vi "display_michelle_visjitter_stopadded_RandCont_PsuedoCO_TSLogFC2.vi"() -> ()   [LabVIEW 2019]
uses:
  <vilib>/Analysis/Matrix/Datatypes/RealMatrix.ctl
  <vilib>/Utility/file.llb/Write Delimited Spreadsheet (DBL).vi
  <vilib>/Analysis/Matrix/NI_Matrix.lvlib
panel:
  out "lambda":dbl
  out "maxITI":dbl
  out "minITI":dbl
  out "goEXP":dbl
  out "meanITI":dbl
  out "Lag1":dbl
  out "TSLog":dbl[][](array[numeric])
  out "TSLog2":dbl[][](array[numeric])
  out "Initialtime":dbl
  out "Time Stamp":timestamp format="%<%H:%M:%S%4u>T"
  out "TSLog1":dbl[][](array[numeric])
  out "ArrayTemp3":T1
  out "StimID2":dbl
  out "Contrast":dbl
  out "TimeOutCounter":i32
  out "ElapsedTime_M":dbl
  out "Base_Contrast":dbl
  out "CurrentTrial":u32=1
  out "Jitter":dbl
  out "BaseITI":dbl
  out "VisStimDuration":dbl
  in  "Stop":bool
  out "Num trials":u32=204
  out "ISI Time":dbl
  out "Stim TS":dbl
  out "Output":dbl[][](array[numeric])
  out "Output frame":T1
  out "Array temp1":T1
  out "Elapsed Time":dbl
  out "Display":bool=TRUE
  out "Trial":u32=1
  out "reward":dbl[](array[numeric])
  out "stim_id":dbl[](array[numeric])
  out "stim_loaded":dbl
  out "Timings":dbl[](array[numeric])
  out "Stimuli Loaded?":bool
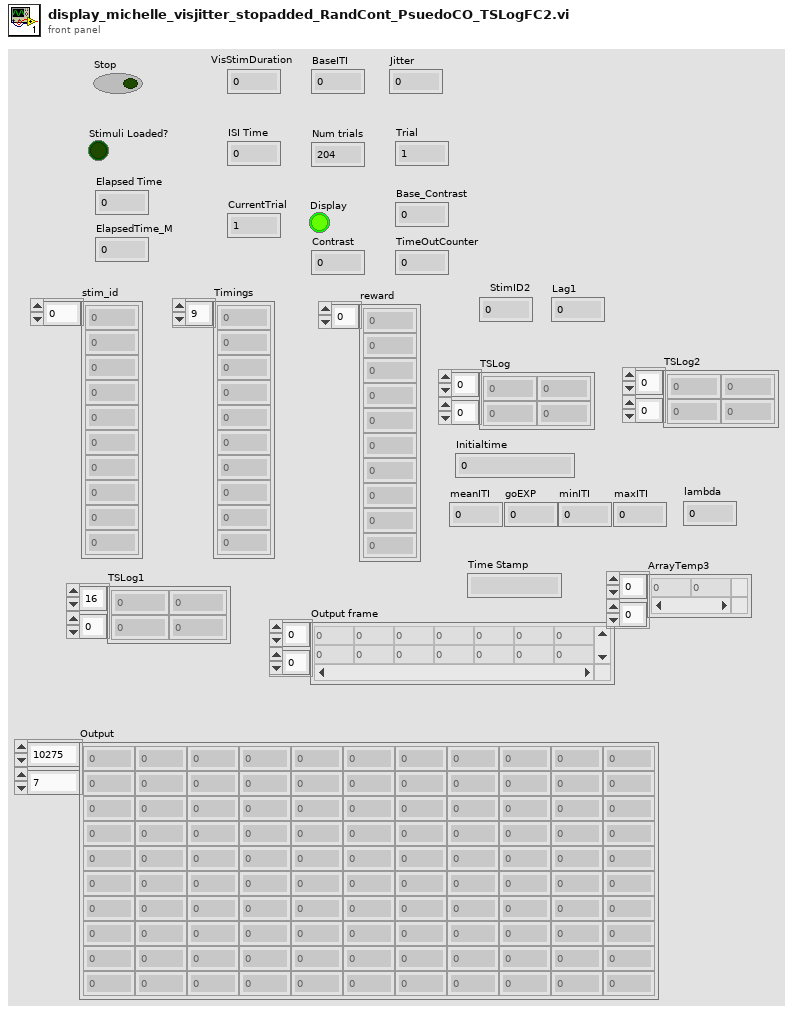
[diagram p1: front panel]
types:
  T1 = typedef "NI_Matrix.lvlib/RealMatrix.ctl" = dbl[][]
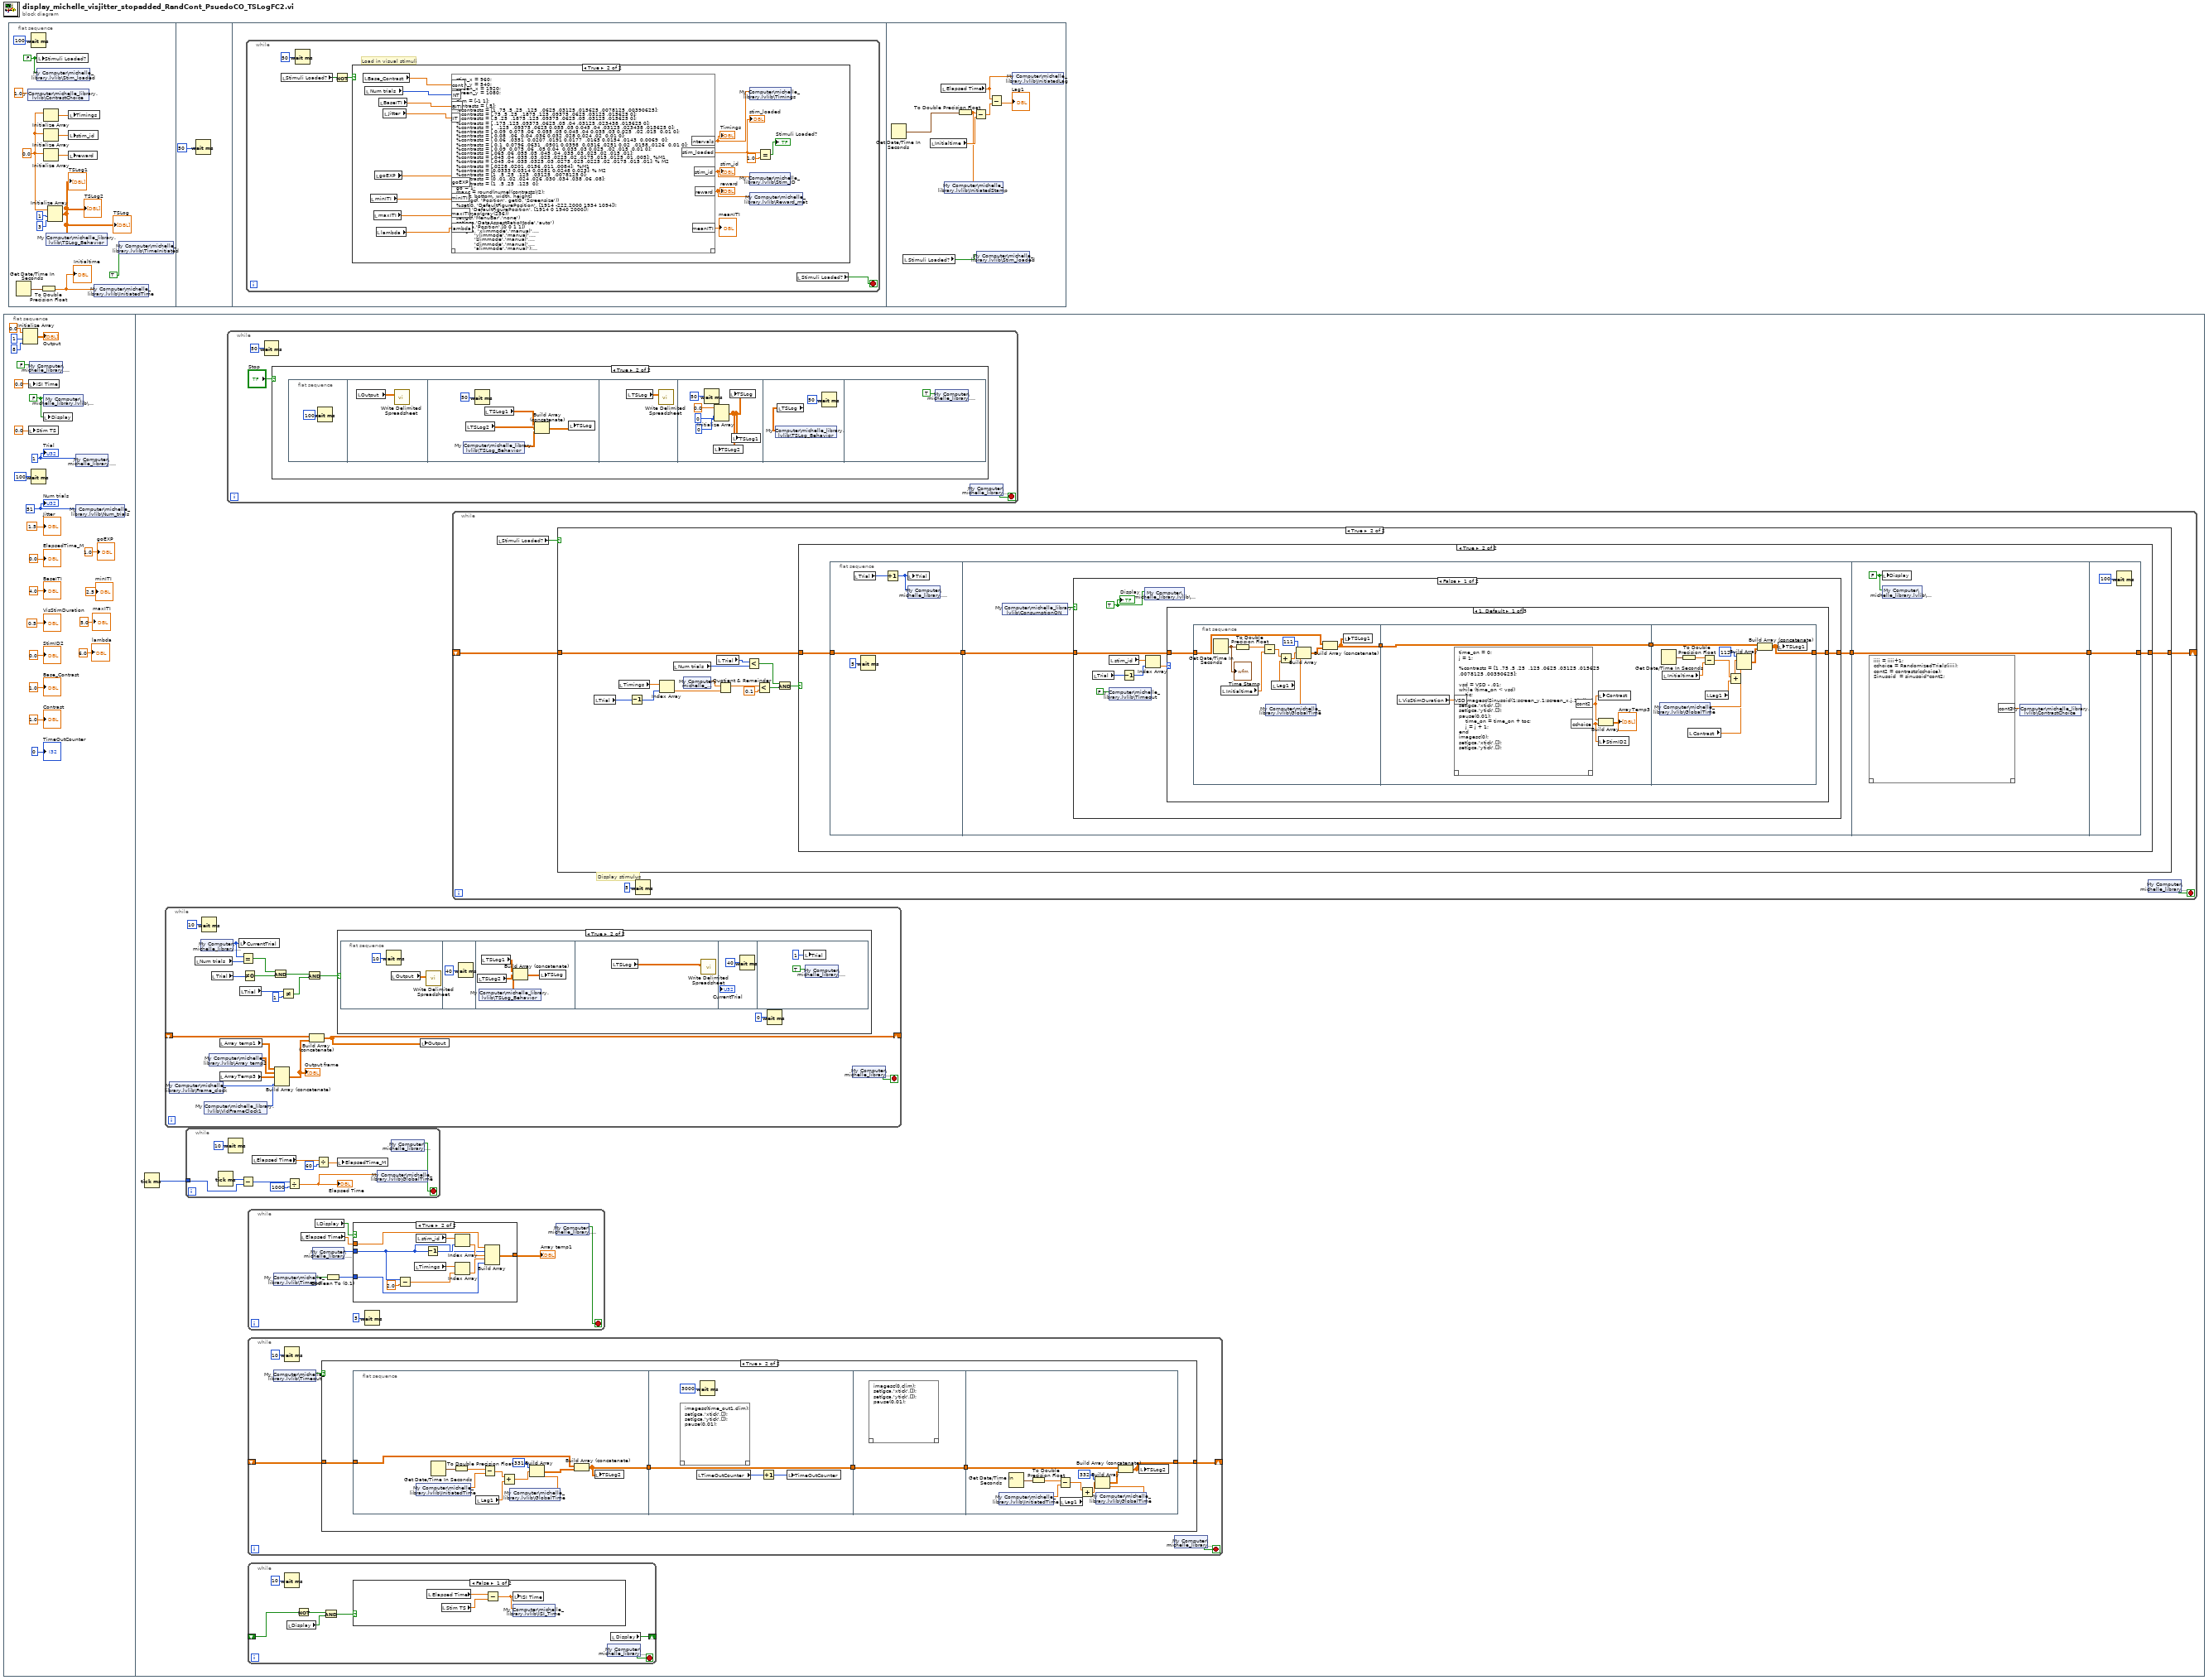
[diagram p0: block diagram]
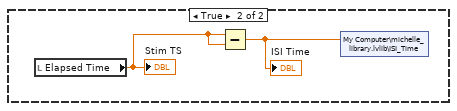
[diagram p5: hidden frame]
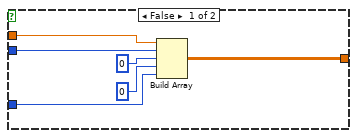
[diagram p6: hidden frame]
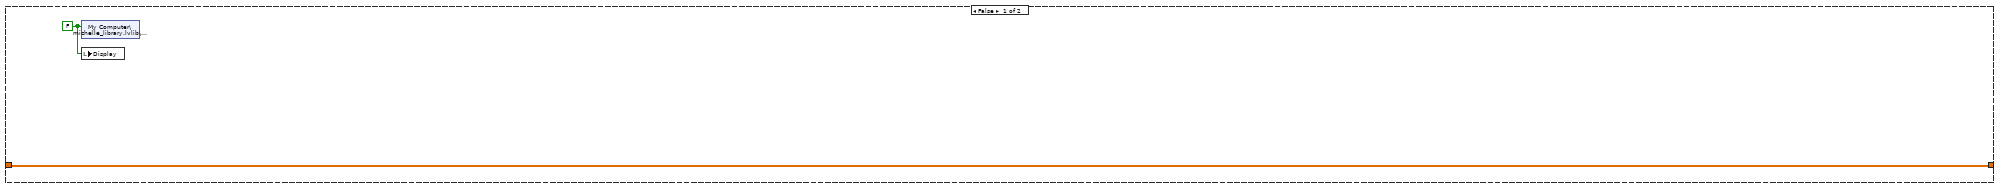
[diagram p9: hidden frame]
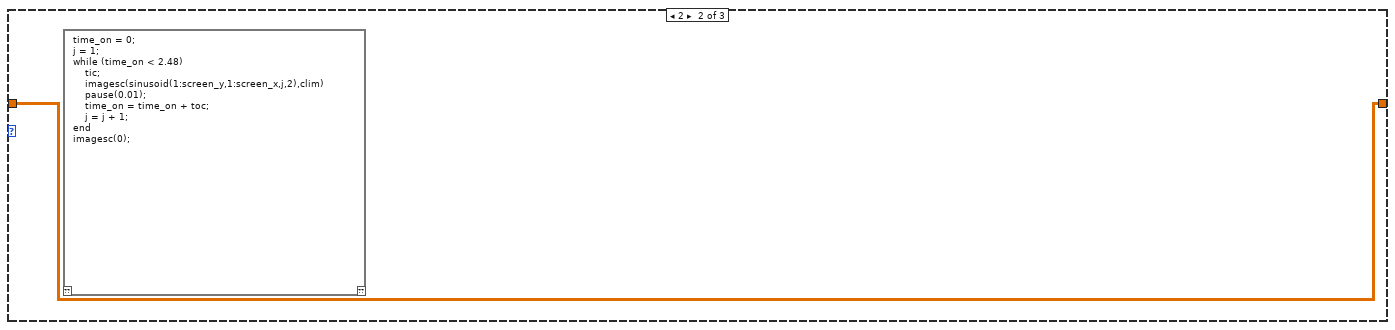
[diagram p10: hidden frame]
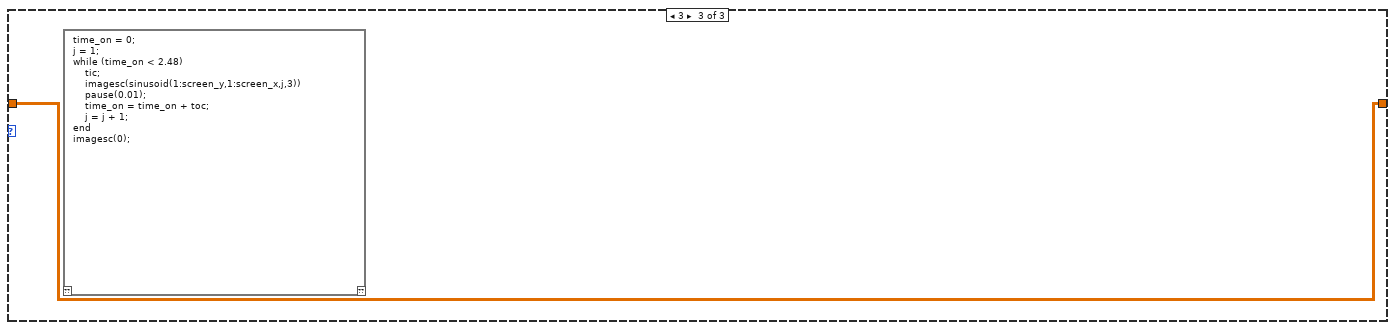
[diagram p11: hidden frame]
diagram:
  n1 = flat-sequence {
    frame #0 {
      w15 = u32 51
      w21 = FALSE ("Display")
      w23 = u32 1 ("Trial")
      n2 = Initialize Array(0.0 ("element"), 1 ("dimension size"), 8 ("dimension size")) -> (→"Output":dbl[][])
      n3 = local write "ISI Time"(0.0 ("ISI Time")) -> ()
      n4 = local write "Stim TS"(0.0 ("Stim TS")) -> ()
      n5 = shared-variable "My Computer\\michelle_library.lvlib\\Stop"(FALSE ("Stop")) -> ()  [unwired: 1 in, 1 out]
      n6 = Wait (ms)(milliseconds to wait=u32 100) -> ()  [unwired: 1 out]
      n7 = shared-variable "My Computer\\michelle_library.lvlib\\Display"(w21) -> ()  [unwired: 1 in, 1 out]
      n8 = local write "Display"(w21) -> ()
      n9 = shared-variable "My Computer\\michelle_library.lvlib\\Trial"(w23) -> ()  [unwired: 1 in, 1 out]
      n10 = shared-variable "My Computer\\michelle_library.lvlib\\Num_trials"(w15) -> ()  [unwired: 1 in, 1 out]
      "Trial" <- w23
      "Num trials" <- w15
      "VisStimDuration" <- 0.5
      "BaseITI" <- 4.0
      "Jitter" <- 1.5
      "Base_Contrast" <- 1.0
      "ElapsedTime_M" <- 0.0
      "TimeOutCounter" <- 0
      "Contrast" <- 1.0
      "StimID2" <- 0.0
      "goEXP" <- 1.0
      "minITI" <- 2.5
      "maxITI" <- 5.0
      "lambda" <- 6.0
    }
    frame #1 {
      n11 = Tick Count (ms)() -> (millisecond timer value=w24:u32)
      n12 = while {
        shift-right: [w145] -> _
        shift-left: _ -> [w146]
        stop <- w148 stop-if-true
        n13 = shared-variable "My Computer\\michelle_library.lvlib\\Frame_clock"() -> (w130:u32)  [unwired: 1 in, 1 out]
        n14 = local read "Num trials"() -> (w141:u32)
        n15 = shared-variable "My Computer\\michelle_library.lvlib\\Trial"() -> (w132:u32)  [unwired: 1 in, 1 out]
        n16 = Wait (ms)(milliseconds to wait=u32 10) -> ()  [unwired: 1 out]
        n17 = shared-variable "My Computer\\michelle_library.lvlib\\VidFrameClock1"() -> (w129:u32)  [unwired: 1 in, 1 out]
        n18 = shared-variable "My Computer\\michelle_library.lvlib\\Array temp2"() -> (w143:dbl[][])  [unwired: 1 in, 1 out]
        n19 = local read "Trial"() -> (w139:u32)
        n20 = local read "Array temp1"() -> (w144:T1)
        n21 = local read "ArrayTemp3"() -> (w131:T1)
        n22 = local write "CurrentTrial"(w132) -> ()
        n23 = local read "Trial"() -> (w138:u32)
        n24 = Equal?(x=w132, y=w141) -> (x = y?=w140:bool)
        n25 = Not Equal To 0?(x=w139) -> (x != 0?=w135:bool)
        n26 = And(x=w140, y=w135) -> (x .and. y?=w133:bool)
        n27 = Build Array (concatenate)(w144, w143, w131, w130, w129) -> (w142:T1)
        "Output frame" <- w142
        n28 = Not Equal?(x=w138, y=1) -> (x != y?=w137:bool)
        n29 = And(x=w133, y=w137) -> (x .and. y?=w134:bool)
        n30 = Build Array (concatenate) ("Build Matrix")(w146, w142) -> (w145:T1)
        n31 = case shown="True" w134 {
          frame False {
          }
          frame True {
            n32 = flat-sequence {
              frame #0 {
                n33 = Wait (ms)(milliseconds to wait=u32 10) -> ()  [unwired: 1 out]
                n34 = local read "Output"() -> (w151:dbl[][])
                n35 = call-poly <vilib>:"Write Delimited Spreadsheet.vi"("2D data"=w151) -> ()  [unwired: 13 in, 2 out]
              }
              frame #1 {
                n36 = Wait (ms)(milliseconds to wait=u32 40) -> ()  [unwired: 1 out]
              }
              frame #2 {
                n37 = local read "TSLog2"() -> (w156:dbl[][])
                n38 = shared-variable "My Computer\\michelle_library.lvlib\\TSLog_Behavior"() -> (w154:dbl[][])  [unwired: 1 in, 1 out]
                n39 = local read "TSLog1"() -> (w155:dbl[][])
                n40 = Build Array (concatenate) ("Build Matrix")(w155, w156, w154) -> (w153:T1)
                n41 = local write "TSLog"(w153) -> ()
              }
              frame #3 {
                n42 = local read "TSLog"() -> (w157:dbl[][])
                n43 = call-poly <vilib>:"Write Delimited Spreadsheet.vi"("2D data"=w157) -> ()  [unwired: 13 in, 2 out]
              }
              frame #4 {
                n44 = Wait (ms)(milliseconds to wait=u32 40) -> ()  [unwired: 1 out]
              }
              frame #5 {
                n45 = local write "Trial"(1) -> ()
                n46 = shared-variable "My Computer\\michelle_library.lvlib\\Stop"(TRUE) -> ()  [unwired: 1 in, 1 out]
              }
            }
            n47 = Wait (ms)(milliseconds to wait=0) -> ()  [unwired: 1 out]
          }
        }
        n48 = local write "Output"(w145) -> ()
        n49 = shared-variable "My Computer\\michelle_library.lvlib\\Stop"() -> (w148:bool)  [unwired: 1 in, 1 out]
      }
      n50 = while {
        tunnel: w24 -> [w126]
        stop <- w123 stop-if-true
        n51 = Tick Count (ms)() -> (millisecond timer value=w127:u32)
        n52 = Wait (ms)(milliseconds to wait=u32 10) -> ()  [unwired: 1 out]
        n53 = Subtract(x=w127, y=w126) -> (x-y=w124:u32)
        n54 = local read "Elapsed Time"() -> (w121:dbl)
        n55 = Divide(x=w124, y=u32 1000) -> (x/y=w119:dbl)
        "Elapsed Time" <- w119
        n56 = Divide(x=w121, y=60) -> (x/y=w120:dbl)
        n57 = local write "ElapsedTime_M"(w120) -> ()
        n58 = shared-variable "My Computer\\michelle_library.lvlib\\GlobalTime"(w119) -> ()  [unwired: 1 in, 1 out]
        n59 = shared-variable "My Computer\\michelle_library.lvlib\\Stop"() -> (w123:bool)  [unwired: 1 in, 1 out]
      }
      n60 = while {
        stop <- w27 stop-if-true
        n61 = Wait (ms)(milliseconds to wait=50) -> ()  [unwired: 1 out]
        n62 = case shown="True" "Stop" {
          frame False {
          }
          frame True {
            n63 = flat-sequence {
              frame #0 {
                n64 = Wait (ms)(milliseconds to wait=100) -> ()  [unwired: 1 out]
              }
              frame #1 {
                n65 = local read "Output"() -> (w29:dbl[][])
                n66 = call-poly <vilib>:"Write Delimited Spreadsheet.vi"("2D data"=w29) -> ()  [unwired: 13 in, 2 out]
              }
              frame #2 {
                n67 = shared-variable "My Computer\\michelle_library.lvlib\\TSLog_Behavior"() -> (w30:dbl[][])  [unwired: 1 in, 1 out]
                n68 = local read "TSLog2"() -> (w33:dbl[][])
                n69 = Wait (ms)(milliseconds to wait=50) -> ()  [unwired: 1 out]
                n70 = local read "TSLog1"() -> (w32:dbl[][])
                n71 = Build Array (concatenate) ("Build Matrix")(w32, w33, w30) -> (w31:T1)
                n72 = local write "TSLog"(w31) -> ()
              }
              frame #3 {
                n73 = local read "TSLog"() -> (w35:dbl[][])
                n74 = call-poly <vilib>:"Write Delimited Spreadsheet.vi"("2D data"=w35) -> ()  [unwired: 13 in, 2 out]
              }
              frame #4 {
                n75 = Wait (ms)(milliseconds to wait=50) -> ()  [unwired: 1 out]
                n76 = Initialize Array(0.0, 0, 0) -> (w37:dbl[][])
                n77 = local write "TSLog2"(w37) -> ()
                n78 = local write "TSLog"(w37) -> ()
                n79 = local write "TSLog1"(w37) -> ()
              }
              frame #5 {
                n80 = local read "TSLog"() -> (w42:dbl[][])
                n81 = shared-variable "My Computer\\michelle_library.lvlib\\TSLog_Behavior"(w42) -> ()  [unwired: 1 in, 1 out]
                n82 = Wait (ms)(milliseconds to wait=50) -> ()  [unwired: 1 out]
              }
              frame #6 {
                n83 = shared-variable "My Computer\\michelle_library.lvlib\\Stop"(TRUE) -> ()  [unwired: 1 in, 1 out]
              }
            }
          }
        }
        n84 = shared-variable "My Computer\\michelle_library.lvlib\\Stop"() -> (w27:bool)  [unwired: 1 in, 1 out]
      }
      n85 = while {
        stop <- w96 stop-if-true
        n86 = shared-variable "My Computer\\michelle_library.lvlib\\Timeout"() -> (w94:bool)  [unwired: 1 in, 1 out]
        n87 = local read "Elapsed Time"() -> (w100:dbl)
        n88 = shared-variable "My Computer\\michelle_library.lvlib\\Trial"() -> (w98:u32)  [unwired: 1 in, 1 out]
        n89 = local read "Display"() -> (w97:bool)
        n90 = Boolean To (0,1)(Boolean=w94) -> (0, 1=w95:i16)
        n91 = case shown="True" w97 {
          tunnel: w98 -> [w106 w109]
          tunnel: w100 -> [w107 w116]
          tunnel: [w105 w117] -> w99
          tunnel: w95 -> [w102 w111]
          frame False {
            n92 = Build Array(w107, w106, u32 0 ("milliseconds to wait"), 0, w102) -> (w105:T1)
          }
          frame True {
            n93 = Subtract(x=w109, y=2.0) -> (x-y=w108:dbl)
            n94 = local read "Timings"() -> (w114:dbl[])
            n95 = local read "stim_id"() -> (w118:dbl[])
            n96 = Decrement(x=w109) -> (x-1=w113:u32)
            n97 = Index Array(array=w118, index=w113) -> (element=w115:dbl)
            n98 = Index Array(array=w114, index=w108) -> (element=w112:dbl)
            n99 = Build Array(w116, w109, w115, w112, w111) -> (w117:T1)
          }
        }
        "Array temp1" <- w99
        n100 = Wait (ms)(milliseconds to wait=u32 5) -> ()  [unwired: 1 out]
        n101 = shared-variable "My Computer\\michelle_library.lvlib\\Stop"() -> (w96:bool)  [unwired: 1 in, 1 out]
      }
      n102 = while {
        shift-right: [w44] -> _
        shift-left: _ -> [w45]
        stop <- w48 stop-if-true
        n103 = shared-variable "My Computer\\michelle_library.lvlib\\Timeout"() -> (w46:bool)  [unwired: 1 in, 1 out]
        n104 = Wait (ms)(milliseconds to wait=u32 10) -> ()  [unwired: 1 out]
        n105 = case shown="True" w46 {
          tunnel: w45 -> [w49 w54]
          tunnel: [w49 w53] -> w44
          frame False {
          }
          frame True {
            n106 = flat-sequence {
              tunnel: w54 -> [w60]
              tunnel: [w59] -> w51
              tunnel: [w66] -> w52
              tunnel: w51 -> [w66]
              tunnel: w52 -> [w70]
              tunnel: [w70] -> w50
              tunnel: [w75] -> w53
              tunnel: w50 -> [w76]
              frame #0 {
                n107 = shared-variable "My Computer\\michelle_library.lvlib\\InitiatedTime"() -> (w63:dbl)  [unwired: 1 in, 1 out]
                n108 = Get Date/Time In Seconds() -> (seconds since 1Jan1904=w65:timestamp)
                n109 = To Double Precision Float(number=w65) -> (double precision float=w64:dbl)
                n110 = local read "Lag1"() -> (w56:dbl)
                n111 = Subtract(x=w64, y=w63) -> (x-y=w57:dbl)
                n112 = Add(x=w57, y=w56) -> (x+y=w58:dbl)
                n113 = shared-variable "My Computer\\michelle_library.lvlib\\GlobalTime"() -> (w55:dbl)  [unwired: 1 in, 1 out]
                n114 = Build Array(331, w58, w55) -> (w62:T1)
                n115 = Build Array (concatenate) ("Build Matrix")(w60, w62) -> (w59:T1)
                n116 = local write "TSLog2"(w59) -> ()
              }
              frame #1 {
                n117 = script code="imagesc(time_out1,clim);\nset(gca,'xtick',[]);\nset(gca,'ytick',[]);\npause(0.01);"() -> ()  [unwired: 1 in, 1 out]
                n118 = local read "TimeOutCounter"() -> (w68:i32)
                n119 = Wait (ms)(milliseconds to wait=u32 3000) -> ()  [unwired: 1 out]
                n120 = Increment(x=w68) -> (x+1=w67:i32)
                n121 = local write "TimeOutCounter"(w67) -> ()
              }
              frame #2 {
                n122 = script code="imagesc(0,clim);\nset(gca,'xtick',[]);\nset(gca,'ytick',[]);\npause(0.01);"() -> ()  [unwired: 1 in, 1 out]
              }
              frame #3 {
                n123 = shared-variable "My Computer\\michelle_library.lvlib\\InitiatedTime"() -> (w81:dbl)  [unwired: 1 in, 1 out]
                n124 = Get Date/Time In Seconds() -> (seconds since 1Jan1904=w79:timestamp)
                n125 = To Double Precision Float(number=w79) -> (double precision float=w80:dbl)
                n126 = Subtract(x=w80, y=w81) -> (x-y=w73:dbl)
                n127 = local read "Lag1"() -> (w72:dbl)
                n128 = Add(x=w73, y=w72) -> (x+y=w74:dbl)
                n129 = shared-variable "My Computer\\michelle_library.lvlib\\GlobalTime"() -> (w71:dbl)  [unwired: 1 in, 1 out]
                n130 = Build Array(332, w74, w71) -> (w77:T1)
                n131 = Build Array (concatenate) ("Build Matrix")(w76, w77) -> (w75:T1)
                n132 = local write "TSLog2"(w75) -> ()
              }
            }
          }
        }
        n133 = shared-variable "My Computer\\michelle_library.lvlib\\Stop"() -> (w48:bool)  [unwired: 1 in, 1 out]
      }
      n134 = while {
        shift-right: [w86] -> _
        shift-left: _ -> [w85]
        stop <- w88 stop-if-true
        n135 = Wait (ms)(milliseconds to wait=u32 10) -> ()  [unwired: 1 out]
        n136 = local read "Display"() -> (w83:bool)
        n137 = Not(x=w85) -> (.not. x?=w84:bool)
        n138 = And(x=w84, y=w83) -> (x .and. y?=w82:bool)
        n139 = case shown="False" w82 {
          frame False {
            n140 = local read "Elapsed Time"() -> (w89:dbl)
            n141 = local read "Stim TS"() -> (w91:dbl)
            n142 = Subtract(x=w89, y=w91) -> (x-y=w90:dbl)
            n143 = local write "ISI Time"(w90) -> ()
            n144 = shared-variable "My Computer\\michelle_library.lvlib\\ISI_Time"(w90) -> ()  [unwired: 1 in, 1 out]
          }
          frame True {
            n145 = local read "Elapsed Time"() -> (w92:dbl)
            "Stim TS" <- w92
            n146 = Subtract(x=w92, y=w92) -> (x-y=w93:dbl)
            "ISI Time" <- w93
            n147 = shared-variable "My Computer\\michelle_library.lvlib\\ISI_Time"(w93) -> ()  [unwired: 1 in, 1 out]
          }
        }
        n148 = shared-variable "My Computer\\michelle_library.lvlib\\Stop"() -> (w88:bool)  [unwired: 1 in, 1 out]
        n149 = local read "Display"() -> (w86:bool)
      }
      n150 = while {
        shift-right: [w161] -> _
        shift-left: _ -> [w162]
        stop <- w164 stop-if-true
        # "Display stimulus"
        n151 = local read "Stimuli Loaded?"() -> (w163:bool)
        n152 = case shown="True" w163 {
          tunnel: w162 -> [w166 w168]
          tunnel: [w166 w167] -> w161
          frame False {
          }
          frame True {
            n153 = local read "Trial"() -> (w169:u32)
            n154 = local read "Timings"() -> (w178:dbl[])
            n155 = Decrement(x=w169) -> (x-1=w170:u32)
            n156 = Index Array(array=w178, index=w170) -> (element=w177:dbl)
            n157 = local read "Num trials"() -> (w173:u32)
            n158 = shared-variable "My Computer\\michelle_library.lvlib\\ISI"() -> (w172:dbl)  [unwired: 1 in, 1 out]
            n159 = local read "Trial"() -> (w176:u32)
            n160 = Quotient & Remainder(x=w172, y=w177) -> (x-y*floor(x/y)=w180:dbl)  [unwired: 1 out]
            n161 = Less?(x=w176, y=w173) -> (x < y?=w175:bool)
            n162 = Less?(x=w180, y=0.1) -> (x < y?=w174:bool)
            n163 = And(x=w175, y=w174) -> (x .and. y?=w171:bool)
            n164 = case shown="True" w171 {
              tunnel: w168 -> [w181 w186]
              tunnel: [w181 w185] -> w167
              frame False {
                w182 = FALSE ("Display")
                n165 = shared-variable "My Computer\\michelle_library.lvlib\\Display"(w182) -> ()  [unwired: 1 in, 1 out]
                n166 = local write "Display"(w182) -> ()
              }
              frame True {
                n167 = flat-sequence {
                  tunnel: [w188] -> w187
                  tunnel: w186 -> [w188]
                  tunnel: w187 -> [w193]
                  tunnel: [w192] -> w183
                  tunnel: [w238] -> w184
                  tunnel: w183 -> [w238]
                  tunnel: [w241] -> w185
                  tunnel: w184 -> [w241]
                  frame #0 {
                    n168 = local read "Trial"() -> (w191:u32)
                    n169 = Wait (ms)(milliseconds to wait=u32 5) -> ()  [unwired: 1 out]
                    n170 = Increment(x=w191) -> (x+1=w190:u32)
                    n171 = local write "Trial"(w190) -> ()
                    n172 = shared-variable "My Computer\\michelle_library.lvlib\\Trial"(w190) -> ()  [unwired: 1 in, 1 out]
                  }
                  frame #1 {
                    n173 = shared-variable "My Computer\\michelle_library.lvlib\\ConsumptionON"() -> (w194:bool)  [unwired: 1 in, 1 out]
                    n174 = case shown="False" w194 {
                      tunnel: w193 -> [w196 w237]
                      tunnel: [w195 w237] -> w192
                      frame False {
                        w197 = TRUE ("Boolean")
                        n175 = local read "Trial"() -> (w200:u32)
                        n176 = shared-variable "My Computer\\michelle_library.lvlib\\Timeout"(FALSE) -> ()  [unwired: 1 in, 1 out]
                        n177 = local read "stim_id"() -> (w202:dbl[])
                        n178 = Decrement(x=w200) -> (x-1=w199:u32)
                        n179 = shared-variable "My Computer\\michelle_library.lvlib\\Display"(w197) -> ()  [unwired: 1 in, 1 out]
                        n180 = Index Array(array=w202, index=w199) -> (element=w201:dbl)
                        n181 = case shown="1, Default" w201 {
                          tunnel: w196 -> [w206 w235 w236]
                          tunnel: [w205 w235 w236] -> w195
                          frame 1, Default {
                            n182 = flat-sequence {
                              tunnel: w206 -> [w216]
                              tunnel: [w215] -> w204
                              tunnel: w204 -> [w218]
                              tunnel: [w218] -> w203
                              tunnel: [w233] -> w205
                              tunnel: w203 -> [w232]
                              frame #0 {
                                n183 = Get Date/Time In Seconds() -> (seconds since 1Jan1904=w213:timestamp)
                                "Time Stamp" <- w213
                                n184 = local read "Initialtime"() -> (w211:dbl)
                                n185 = To Double Precision Float(number=w213) -> (double precision float=w212:dbl)
                                n186 = Subtract(x=w212, y=w211) -> (x-y=w209:dbl)
                                n187 = shared-variable "My Computer\\michelle_library.lvlib\\GlobalTime"() -> (w207:dbl)  [unwired: 1 in, 1 out]
                                n188 = local read "Lag1"() -> (w210:dbl)
                                n189 = Add(x=w209, y=w210) -> (x+y=w208:dbl)
                                n190 = Build Array(111, w208, w207) -> (w214:T1)
                                n191 = Build Array (concatenate) ("Build Matrix")(w216, w214) -> (w215:T1)
                                n192 = local write "TSLog1"(w215) -> ()
                              }
                              frame #1 {
                                n193 = local read "VisStimDuration"() -> (w220:dbl)
                                n194 = script code="time_on = 0;\nj = 1;\n\n%contrasts = [1 .75 .5 .25  .125 .0625 .03125 .015625 .0078125 .00390625];\n\nvsd = VSD - .01;\nwhile (time_on < vsd)\n    tic;\n    imagesc(Sinusoid(1:screen_y,1:screen_x,j,1),clim)\nset(gca,'xtick',[]);\nset(gca,'ytick',[]);    \npause(0.01);\n    time_on = time_on + toc;\n    j = j + 1;\nend\nimagesc(0);\nset(gca,'xtick',[]);\nset(gca,'ytick',[]);"("VSD"=w220) -> ("cont2"=w222:dbl, "cchoice"=w221:dbl)  [unwired: 1 in, 1 out]
                                n195 = local write "Contrast"(w222) -> ()
                                n196 = Build Array(w222, w221) -> (→"ArrayTemp3":T1)
                                n197 = local write "StimID2"(w221) -> ()
                              }
                              frame #2 {
                                n198 = shared-variable "My Computer\\michelle_library.lvlib\\GlobalTime"() -> (w224:dbl)  [unwired: 1 in, 1 out]
                                n199 = Get Date/Time In Seconds() -> (seconds since 1Jan1904=w230:timestamp)
                                n200 = local read "Initialtime"() -> (w229:dbl)
                                n201 = To Double Precision Float(number=w230) -> (double precision float=w228:dbl)
                                n202 = local read "Contrast"() -> (w223:dbl)
                                n203 = Subtract(x=w228, y=w229) -> (x-y=w227:dbl)
                                n204 = local read "Lag1"() -> (w225:dbl)
                                n205 = Add(x=w227, y=w225) -> (x+y=w226:dbl)
                                n206 = Build Array(112, w226, w224, w223) -> (w234:T1)
                                n207 = Build Array (concatenate) ("Build Matrix")(w232, w234) -> (w233:T1)
                                n208 = local write "TSLog1"(w233) -> ()
                              }
                            }
                          }
                          frame 2 {
                            n209 = script code="time_on = 0;\nj = 1;\nwhile (time_on < 2.48)\n    tic;\n    imagesc(sinusoid(1:screen_y,1:screen_x,j,2),clim)\n    pause(0.01);\n    time_on = time_on + toc;\n    j = j + 1;\nend\nimagesc(0);"() -> ()  [unwired: 1 in, 1 out]
                          }
                          frame 3 {
                            n210 = script code="time_on = 0;\nj = 1;\nwhile (time_on < 2.48)\n    tic;\n    imagesc(sinusoid(1:screen_y,1:screen_x,j,3))\n    pause(0.01);\n    time_on = time_on + toc;\n    j = j + 1;\nend\nimagesc(0);"() -> ()  [unwired: 1 in, 1 out]
                          }
                        }
                        "Display" <- w197
                      }
                      frame True {
                      }
                    }
                  }
                  frame #2 {
                    w240 = FALSE ("Display")
                    n211 = script code="iiii = iiii+1;\ncchoice = RandomizedTrials(iiii);\ncont2 = contrasts(cchoice);\nSinusoid  = sinusoid*cont2;"() -> ("cont2"=w239:dbl)  [unwired: 1 in, 1 out]
                    n212 = local write "Display"(w240) -> ()
                    n213 = shared-variable "My Computer\\michelle_library.lvlib\\Display"(w240) -> ()  [unwired: 1 in, 1 out]
                    n214 = shared-variable "My Computer\\michelle_library.lvlib\\ContrastChoice"(w239) -> ()  [unwired: 1 in, 1 out]
                  }
                  frame #3 {
                    n215 = Wait (ms)(milliseconds to wait=u32 100) -> ()  [unwired: 1 out]
                  }
                }
              }
            }
          }
        }
        n216 = Wait (ms)(milliseconds to wait=u32 5) -> ()  [unwired: 1 out]
        n217 = shared-variable "My Computer\\michelle_library.lvlib\\Stop"() -> (w164:bool)  [unwired: 1 in, 1 out]
      }
    }
  }
  n218 = flat-sequence {
    frame #0 {
      w249 = 0.0 ("element")
      w251 = FALSE ("Stimuli Loaded?")
      n219 = Get Date/Time In Seconds() -> (seconds since 1Jan1904=w246:timestamp)
      n220 = shared-variable "My Computer\\michelle_library.lvlib\\ContrastChoice"(1.0) -> ()  [unwired: 1 in, 1 out]
      n221 = Wait (ms)(milliseconds to wait=u32 100) -> ()  [unwired: 1 out]
      n222 = local write "Stimuli Loaded?"(w251) -> ()
      n223 = shared-variable "My Computer\\michelle_library.lvlib\\Stim_loaded"(w251) -> ()  [unwired: 1 in, 1 out]
      n224 = To Double Precision Float(number=w246) -> (double precision float=w245:dbl)
      "Initialtime" <- w245
      n225 = Initialize Array(w249) -> (w254:dbl[])  [unwired: 1 in]
      n226 = Initialize Array(w249) -> (w253:dbl[])  [unwired: 1 in]
      n227 = Initialize Array(w249) -> (w252:dbl[])  [unwired: 1 in]
      n228 = Initialize Array(w249, 1, 3) -> (w243:dbl[][])
      "TSLog1" <- w243
      "TSLog2" <- w243
      "TSLog" <- w243
      n229 = shared-variable "My Computer\\michelle_library.lvlib\\TSLog_Behavior"(w243) -> ()  [unwired: 1 in, 1 out]
      n230 = local write "Timings"(w254) -> ()
      n231 = local write "stim_id"(w253) -> ()
      n232 = local write "reward"(w252) -> ()
      n233 = shared-variable "My Computer\\michelle_library.lvlib\\InitiatedTime"(w245) -> ()  [unwired: 1 in, 1 out]
      n234 = shared-variable "My Computer\\michelle_library.lvlib\\TimeInitiated"(TRUE) -> ()  [unwired: 1 in, 1 out]
    }
    frame #1 {
      n235 = Wait (ms)(milliseconds to wait=u32 50) -> ()  [unwired: 1 out]
    }
    frame #2 {
      n236 = while {
        stop <- w257 stop-if-true
        # "Load in visual stimuli"
        n237 = local read "Stimuli Loaded?"() -> (w259:bool)
        n238 = Wait (ms)(milliseconds to wait=u32 50) -> ()  [unwired: 1 out]
        n239 = Not(x=w259) -> (.not. x?=w258:bool)
        n240 = case shown="True" w258 {
          frame False {
          }
          frame True {
            n241 = local read "Base_Contrast"() -> (w267:dbl)
            n242 = local read "Num trials"() -> (w270:u32)
            n243 = local read "minITI"() -> (w263:dbl)
            n244 = local read "maxITI"() -> (w262:dbl)
            n245 = local read "goEXP"() -> (w264:dbl)
            n246 = local read "lambda"() -> (w261:dbl)
            n247 = local read "BaseITI"() -> (w269:dbl)
            n248 = local read "Jitter"() -> (w268:dbl)
            n249 = script code="stim_x = 960;\nstim_y = 540;\nscreen_x = 1920;\nscreen_y = 1080;\n\nclim = [-1 1];\ncontrasts = [.5];\n%contrasts = [1 .75 .5 .25  .125  .0625 .03125 .015625 .0078125 .00390625];\n%contrasts = [.75 .5 .25  .1875 .125 .09375 .0625 .03125 .015625 0];\n%contrasts = [.5 .25  .1875 .125 .09375 .0625 .05 .03125 .015625 0];\n%contrasts = [ .175 .125 .09375 .0625 .05 .04 .03125 .023438 .015625 0];\n%contrasts = [   .125  .09375 .0625 0.055 .05 0.045 .04 .03125 .023438 .015625 0];\n%contrasts = [ 0.09  0.075 .06  0.055 .05 0.045 .04 0.035 .03 0.025  .02 .015  0.01 0];\n%contrasts = [ 0.08  .06  0.04 .036 0.032 .028 0.024 .02  0.01 0];\n%contrasts = [ 0.06  .0351  0.0207 .0191 0.0177  .0165 0.0154 .0143  0.0069  0];\n%contrasts = [ 0.1  0.0796 .0631  .0501 0.0398  0.0316 .0251 0.02  .0158 .0126  0.01 0];\n%contrasts = [ 0.09  0.075 .06  .05 0.04  0.035 .03 0.025  .02 .015  0.01 0];\n%contrasts = [.065 .06 .055 .05 .045 .04 .035 .03 .025 .02 .015 .01];\n%contrasts = [.045 .04 .035 .03 .025 .0225 .02 .0175 .015 .0125 .01 .005];  %M1\n%contrasts = [.045 .04 .035 .0325 .03 .0275 .025 .0225 .02 .0175 .015 .01]; % M2\n%contrasts = [.0228 .0201 .0156 .011 .0084];  %M1\n%contrasts = [0.0333 0.0314 0.0281 0.0248 0.023]; % M2\n%contrasts = [1  .5 .25  .125  .03125  .0078125 0];\n%contrasts = [0 .01 .02 .024 .026 .030 .034 .038 .06 .08];\n%contrasts = [1  .5 .25  .125  0];\ngo = 1;\nmaxc = round(numel(contrasts)/2);\n%[left, bottom, width, height]\n%set(gcf, 'Position', get(0, 'Screensize'))\n%set(0, 'DefaultFigurePosition', [1914 -222.2000 1934 1094]);\nset(0, 'DefaultFigurePosition', [1914 0 1940 2000]);\ncolormap(gray(256))\nset(gcf,'MenuBar','none')\nset(gca,'DataAspectRatioMode','auto')\nset(gca,'Position',[0 0 1 1])\nset(gca, 'xlimmode','manual',...\n           'ylimmode','manual',...\n           'zlimmode','manual',...\n           'climmode','manual',...\n           'alimmode','manual');\n\nimagesc(0);\nset(gca,'xtick',[]);\nset(gca,'ytick',[]);\npause(0.01);\n\n% Define grating parameters\norientation = [14*pi/18; 13*pi/18];\n\ncenter = [1,1]; %[0,0] is the middle of the image, [pi,pi] is the lower right\n%width = .5;  %1/e half width of Gaussian\nspatialFrequency = 8;  %spatial frequency of Sinewave carrier (cycles/image)\nphase = -pi/2; %spatial phase of sinewave carrier (radians)\ncontrast = cont;  %contrast ranges from 0 to 1;\n%screen_x = 1920; %resolution of the image  \n%screen_y = 1080;\n\n% Use meshgrid to define matrices X and Y that range from -pi to pi;\n[X,Y] = meshgrid(linspace(-pi,pi,screen_x),linspace(-pi/2,pi/2,screen_y));\n\nsinusoid = zeros(screen_y,screen_x,150,2);\ntime_out1 = ones(screen_y,screen_x)*-1;\ntime_out2 = zeros(screen_y,screen_x);\n%time_out(1,1) = 1;\n% Set up individual 4-d matrices (x, y, time, orientation) for movies of the drifting gratings at each\n% orientation\nfor j = 1:length(orientation)                                                            % Phase increase number here\n    ramp(1:screen_y,1:screen_x,j) = cos(orientation(j))*(X-center(1)) + sin(orientation(j))*(Y-center(2));     %  |\n    for i = 1:150 %Sets the number of frames to define gratings for                   V\n       sinusoid(1:screen_y,1:screen_x,i,j) = contrast*sin(spatialFrequency*ramp(1:screen_y,1:screen_x,j)-...\n           (phase+(2*pi*(i-1)*(-30)/360))); %Number before '/360' sets the phase increase\n    end\nend\n\n\n\n[RandomizedTrials]=RandomizeTrials_Psuedo_function(contrasts,NT,'n');\n\n\niiii = 1;\n\ncchoice = RandomizedTrials(iiii);\ncont2 = contrasts(cchoice);\nSinusoid  = sinusoid*cont2;\n\n\n%%  To be run of not using exponential\n%intervals = [ones(1,41)*10 ones(1,41)*11 ones(1,41)*12 ones(1,41)*13 ones(1,40)*14];\nif goEXP < 1\n     jit = JIT;\n     jitter = rand(1,NT);\n     jitter = 2*jit*(jitter- .5);\n     ITIbase = BITI;\n     intervals = [ones(1,NT)*ITIbase];\n     intervals = intervals + jitter;\nelseif goEXP > 0\n     intervals = exponentialITI(1/lambda, minITI, maxITI, NT);\nend\n%%\nstim_id = [ones(1,NT)*1];\n%reward = [ones(1,87)*1 ones(1,15)*0 ones(1,87)*1 ones(1,15)*0];\nreward = [ones(1,NT)*1];\nmeanITI = nanmean(intervals);\n\n\nrand_idx1 = randperm(NT);\nrand_idx2 = randperm(NT);\nintervals = intervals(rand_idx2);\nstim_id = stim_id(rand_idx2);\nreward = reward(rand_idx2);\n\nstim_loaded = 1;" ("Script Node")("NT"=w270, "BITI"=w269, "JIT"=w268, "cont"=w267, "goEXP"=w264, "minITI"=w263, "maxITI"=w262, "lambda"=w261) -> ("stim_loaded"=w275:dbl, "intervals"=w271:dbl[], "stim_id"=w272:dbl[], "reward"=w273:dbl[], "meanITI"=→"meanITI":dbl)  [unwired: 1 in, 1 out]
            "stim_loaded" <- w275
            "Timings" <- w271
            "stim_id" <- w272
            "reward" <- w273
            n250 = shared-variable "My Computer\\michelle_library.lvlib\\Timings"(w271) -> ()  [unwired: 1 in, 1 out]
            n251 = shared-variable "My Computer\\michelle_library.lvlib\\Stim_ID"(w272) -> ()  [unwired: 1 in, 1 out]
            n252 = shared-variable "My Computer\\michelle_library.lvlib\\Reward_mat"(w273) -> ()  [unwired: 1 in, 1 out]
            n253 = Equal?(x=w275, y=1.0) -> (x = y?=→"Stimuli Loaded?":bool)
          }
        }
        n254 = local read "Stimuli Loaded?"() -> (w257:bool)
      }
    }
    frame #3 {
      n255 = Get Date/Time In Seconds() -> (seconds since 1Jan1904=w282:timestamp)
      n256 = local read "Stimuli Loaded?"() -> (w277:bool)
      n257 = local read "Initialtime"() -> (w281:dbl)
      n258 = local read "Elapsed Time"() -> (w276:dbl)
      n259 = To Double Precision Float(number=w282) -> (double precision float=w279:dbl)
      n260 = shared-variable "My Computer\\michelle_library.lvlib\\InitiatedStamp"(w279) -> ()  [unwired: 1 in, 1 out]
      n261 = Subtract(x=w279, y=w281) -> (x-y=w280:dbl)
      n262 = shared-variable "My Computer\\michelle_library.lvlib\\Stim_loaded"(w277) -> ()  [unwired: 1 in, 1 out]
      n263 = Subtract(x=w276, y=w280) -> (x-y=→"Lag1":dbl)
      n264 = shared-variable "My Computer\\michelle_library.lvlib\\InitiatedLag"(w276) -> ()  [unwired: 1 in, 1 out]
    }
  }
